vi "ResizeMulticolCol1.vi"(8 "error in (no error)":errorcluster, 11 "MulticolumnListbox in":refnum<vi>) -> (0 "error out":errorcluster, 3 "MulticolumnListbox out":refnum<vi>)   [LabVIEW 2017]
uses:
  <vilib>/Utility/miscctls.llb/LVRowAndColumnTypeDef.ctl
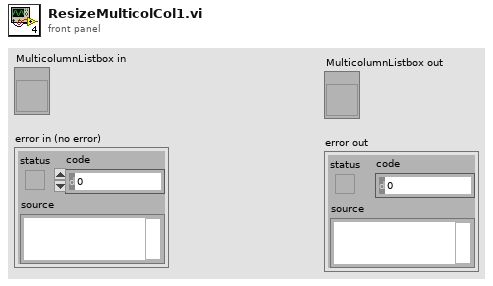
[diagram p1: front panel]
types:
  T1 = typedef "LVRowAndColumnTypeDef.ctl" = cluster{"Row":i32, "Column":i32}
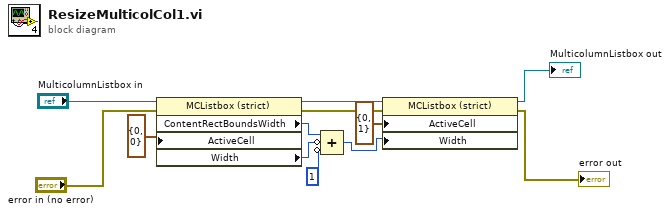
[diagram p0: block diagram]
diagram:
  n1 = property class="MCListbox (strict)"(reference="MulticolumnListbox in", error in="error in (no error)", "ActiveCell"=T1 {"Row"=0, "Column"=0} ("Active Cell:Active Cell")) -> (reference out=w9:refnum<vi>, error out=w8:errorcluster, "ContentRectBoundsWidth"=w5:i32, "Width"=w6:u32)
  n2 = Compound Arithmetic op=ADD(w5, invert w6, invert u32 1 ("value")) -> (w4:u32)
  n3 = property class="MCListbox (strict)"(reference=w9, error in=w8, "ActiveCell"=T1 {"Row"=0, "Column"=1} ("Active Cell:Active Cell"), "Width"=w4) -> (reference out=→"MulticolumnListbox out":refnum<vi>, error out=→"error out":errorcluster)
